vi "Handle State.vi"(8 "error in (no error)":errorcluster, 9 "Sender":refnum<class "Message Enqueuer.lvclass">, 10 "Process State":T1, 11 "ProcStateHandler in":refnum<class "ProcStateHandler.lvclass">) -> (0 "error out":errorcluster, 3 "ProcStateHandler out":refnum<class "ProcStateHandler.lvclass">)   [LabVIEW 2020, in "LAF2024Q2.lvlib" / "ProcStateHandler.lvclass"]
uses:
  ProcStateHandler.lvclass
  Process State.ctl
  <vilib>/ActorFramework/Message Enqueuer/Message Enqueuer.lvclass
  LAF2024Q2.lvlib
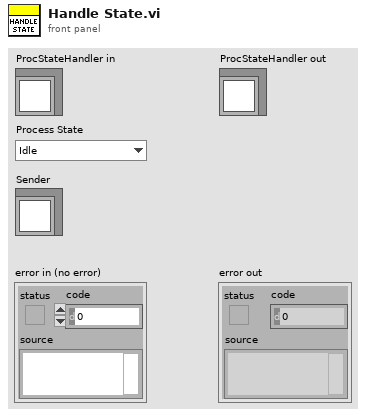
[diagram p1: front panel]
types:
  T1 = typedef "LAF2024Q2.lvlib/Process State.ctl" = enum16{"Idle", "Initializing", "Starting", "Running", "Stopping", "Stopped"}
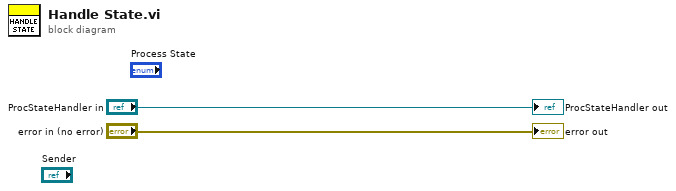
[diagram p0: block diagram]
diagram:
  "error out" <- "error in (no error)"
  "ProcStateHandler out" <- "ProcStateHandler in"
